vi "Link Transmit Parameters.vi"(7 "Parameter R Table in":refnum<class "Registry.lvclass">, 8 "error in (no error)":errorcluster, 11 "Message in":refnum<class "Message.lvclass">) -> (0 "error out":errorcluster, 5 "Parameter R Table out":refnum<class "Registry.lvclass">)   [LabVIEW 2020, in "BCI-1553 API.lvlib" / "Message.lvclass"]
doc: "<DO NOT CALL>\n\nIf this is a transmit message, we take all the parameters and add them to the parameter read table."
uses:
  Message.lvclass
  Dependencies/Registry/Registry.lvclass
  TypeDefs/Command Type.ctl
  Message.lvclass/Message.ctl
  Dependencies/Registry/Registry.lvclass/Registry.ctl
  BCI-1553 API.lvlib
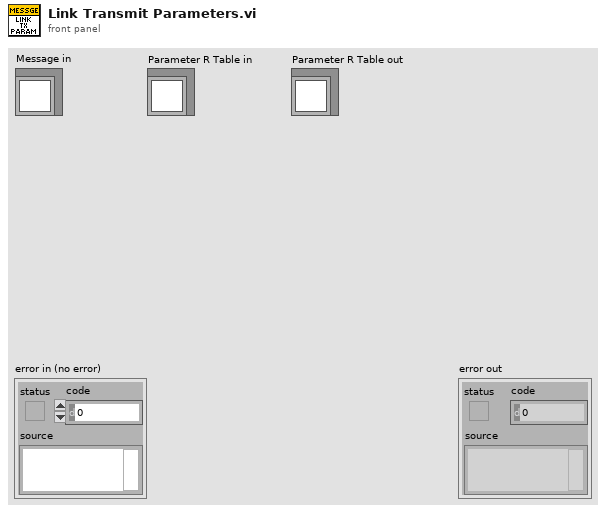
[diagram p1: front panel]
types:
  T1 = typedef "BCI-1553 API.lvlib/Command Type.ctl" = enum16{"Transmit", "Receive"}
  T2 = typedef "BCI-1553 API.lvlib/Parameter Table Data.ctl" = cluster{"Parameter Name":string, "Base Word":u16, "Address":u16, "Value":u64, "Mask":u16[], "Scaling Info":T3}
  T3 = typedef "BCI-1553 API.lvlib/Scaling Information.ctl" = cluster{"Bit Offset":i32, "Bit Count":i32, "LSB Resolution":dbl, "2's Complement":bool, "Big Endian":bool, "Sign Bit":bool}
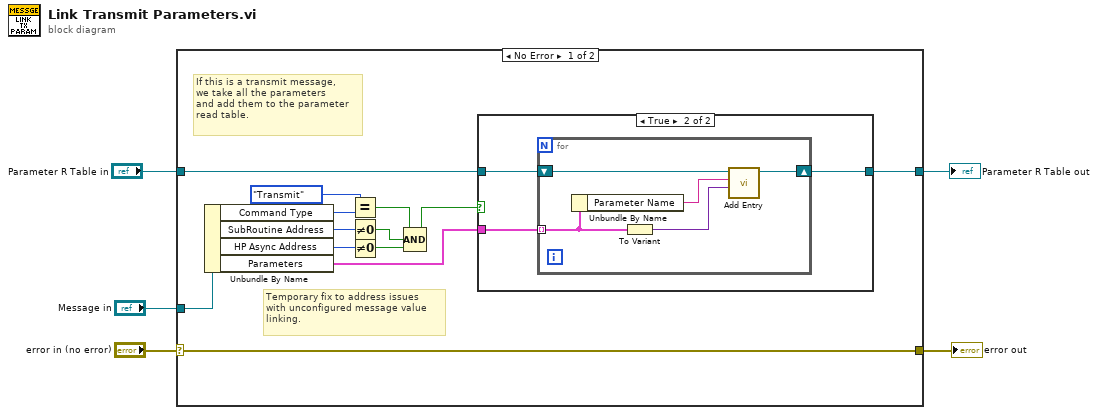
[diagram p0: block diagram]
diagram:
  n1 = case shown="No Error" "error in (no error)" {
    selector: "error in (no error)" -> [w18 w29]
    tunnel: [w18 w29] -> w3
    tunnel: "Message in" -> [w15 _]
    tunnel: "Parameter R Table in" -> [w17 w28]
    tunnel: [w16 w28] -> w1
    frame No Error {
      # "Temporary fix to address issues\nwith unconfigured message value\nlinking."
      # "If this is a transmit message,\nwe take all the parameters\nand add them to the parameter\nread table."
      n2 = Unbundle By Name(w15) -> ("Command Type"=w14:T1, "SubRoutine Address"=w11:u16, "HP Async Address"=w7:u16, "Parameters"=w13:T2[])
      n3 = Equal?(x=Command_Type."Transmit", y=w14) -> (x = y?=w9:bool)
      n4 = Not Equal To 0?(x=w11) -> (x != 0?=w10:bool)
      n5 = Not Equal To 0?(x=w7) -> (x != 0?=w6:bool)
      n6 = Compound Arithmetic op=AND(w9, w10, w6) -> (w8:bool)
      n7 = case shown="True" w8 {
        tunnel: w17 -> [w19 w22]
        tunnel: [w19 w21] -> w16
        tunnel: w13 -> [_ w20]
        frame False {
        }
        frame True {
          n8 = for {
            shift-right: [w26] -> w21
            shift-left: w22 -> [w27]
            tunnel: w20 -> [w25] mode=indexing
            n9 = Unbundle By Name(w25) -> ("Parameter Name"=w23:string)
            n10 = To Variant(anything=w25) -> (Variant=w24:variant)
            n11 = call "Add Entry.vi"("Value"=w24, "Key"=w23, "Registry in"=w27) -> ("Registry out"=w26:refnum<class "Registry.lvclass">)  [unwired: 6 in, 2 out]
          }
        }
      }
    }
    frame Error {
    }
  }
  "error out" <- w3
  "Parameter R Table out" <- w1
